vi "Init.vi"(7 "Enclave":refnum<class "Enclave.lvclass">) -> (3 "Writer out":refnum<class "Writer.lvclass">)   [LabVIEW 2022 SP3, in "Enclave.lvlib" / "Writer.lvclass"]
uses:
  Writer.lvclass
  Enclave/Enclave.lvclass
  Writer.lvclass/Writer.ctl
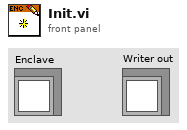
[diagram p1: front panel]
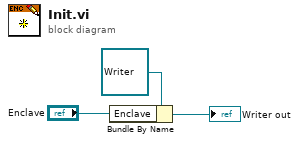
[diagram p0: block diagram]
diagram:
  n1 = Bundle By Name(cluster=refnum<class "Writer.lvclass"> refnum ("Writer in"), "Enclave"="Enclave") -> (→"Writer out":refnum<class "Writer.lvclass">)
